vi "State Enter Core.vi"(8 "error in (no error)":errorcluster, 11 "B Context State in":refnum<class "B Context State.lvclass">) -> (0 "error out":errorcluster, 3 "B Context State out":refnum<class "B Context State.lvclass">)   [LabVIEW 2021, in "Context.lvlib" / "B Context State.lvclass"]
uses:
  B Context State.lvclass
  B Context State.lvclass/B Context State.ctl
  Context/Context.lvclass
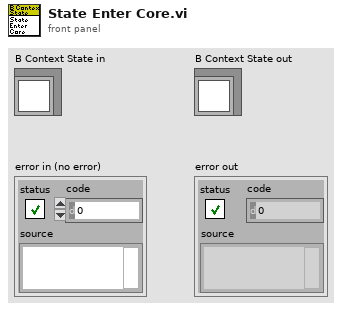
[diagram p1: front panel]
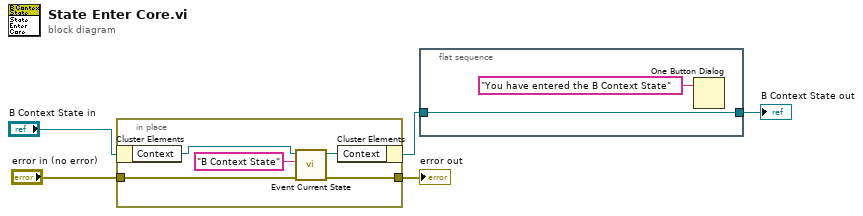
[diagram p0: block diagram]
diagram:
  n1 = in-place {
    in-place-border: "error in (no error)" -> [w8]
    in-place-border: [w7] -> w4
    n2 = in-place-cluster #1("B Context State in") -> ("Context"=w10:refnum<class "Context.lvclass">)
    n3 = call "Event Current State.vi"("error in (no error)"=w8, "Current State"="B Context State", "Context in"=w10) -> ("error out"=w7:errorcluster, "Context out"=w9:refnum<class "Context.lvclass">)  [unwired: 7 in]
    n4 = in-place-cluster #1("Context"=w9) -> (w1:refnum<class "B Context State.lvclass">)
  }
  "error out" <- w4
  n5 = flat-sequence {
    tunnel: [w11] -> w5
    tunnel: w1 -> [w11]
    frame #0 {
      n6 = One Button Dialog(message="You have entered the B Context State") -> ()  [unwired: 1 in, 1 out]
    }
  }
  "B Context State out" <- w5
